vi "execute.vi"(8 "error in (no error)":errorcluster, 9 "ParameterString":string, 10 "ObjectCluster":T1, 11 "RoomLightCommand in":refnum<class "RoomLightCommand.lvclass">) -> (0 "error out":errorcluster, 2 "ObjectCluster Out":T1, 3 "RoomLightCommand out":refnum<class "RoomLightCommand.lvclass">)   [LabVIEW 2013, in "RoomLightCommand.lvclass"]
uses:
  RoomLightCommand.lvclass
  Command.lvclass/ObjectCluster.ctl
  AirCondition.lvclass/AirCondition.lvclass
  RoomLight.lvclass/RoomLight.lvclass
  OutDoorLight.lvclass/OutDoorLight.lvclass
  Television.lvclass/Television.lvclass
  Stereo.lvclass/Stereo.lvclass
  Command.lvclass/Command.lvclass
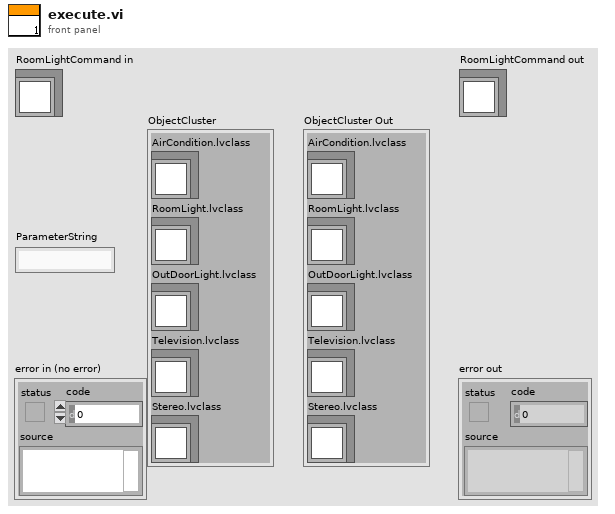
[diagram p1: front panel]
types:
  T1 = typedef "Command.lvclass/ObjectCluster.ctl" = cluster{"AirCondition.lvclass":refnum<class "AirCondition.lvclass">, "RoomLight.lvclass":refnum<class "RoomLight.lvclass">, "OutDoorLight.lvclass":refnum<class "OutDoorLight.lvclass">, "Television.lvclass":refnum<class "Television.lvclass">, "Stereo.lvclass":refnum<class "Stereo.lvclass">}
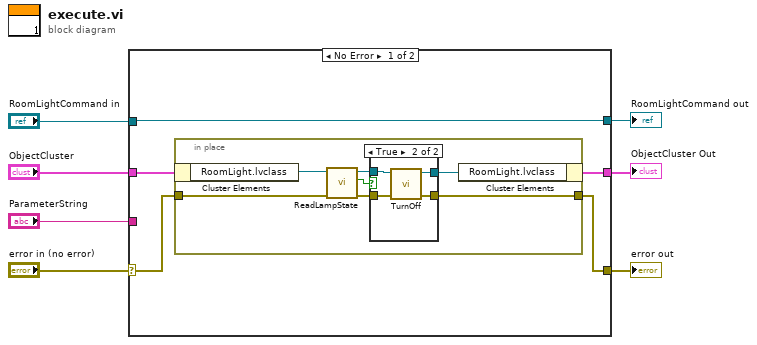
[diagram p0: block diagram]
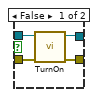
[diagram p2: hidden frame]
diagram:
  n1 = case shown="No Error" "error in (no error)" {
    selector: "error in (no error)" -> [w11 w28]
    tunnel: "ObjectCluster" -> [w12 w29]
    tunnel: "RoomLightCommand in" -> [w8 w30]
    tunnel: "ParameterString" -> [_ _]
    tunnel: [w10 w28] -> w3
    tunnel: [w9 w29] -> w2
    tunnel: [w8 w30] -> w1
    frame No Error {
      n2 = in-place {
        in-place-border: w11 -> [w14]
        in-place-border: [w13] -> w10
        n3 = in-place-cluster #1(w12) -> ("RoomLight.lvclass"=w16:refnum<class "RoomLight.lvclass">)
        n4 = call-dynamic "ReadLampState.vi"("error in (no error)"=w14, "RoomLight in"=w16) -> ("error out"=w17:errorcluster, "LampState"=w19:bool, "RoomLight out"=w18:refnum<class "RoomLight.lvclass">)  [unwired: 7 in]
        n5 = case shown="True" w19 {
          tunnel: w18 -> [w23 w27]
          tunnel: w17 -> [w21 w26]
          tunnel: [w22 w25] -> w15
          tunnel: [w20 w24] -> w13
          frame False {
            n6 = call-dynamic "TurnOn.vi"("error in (no error)"=w21, "RoomLight in"=w23) -> ("error out"=w20:errorcluster, "RoomLight out"=w22:refnum<class "RoomLight.lvclass">)  [unwired: 8 in]
          }
          frame True {
            n7 = call-dynamic "TurnOff.vi"("error in (no error)"=w26, "RoomLight in"=w27) -> ("error out"=w24:errorcluster, "RoomLight out"=w25:refnum<class "RoomLight.lvclass">)  [unwired: 8 in]
          }
        }
        n8 = in-place-cluster #1("RoomLight.lvclass"=w15) -> (w9:T1)
      }
    }
    frame Error {
    }
  }
  "error out" <- w3
  "RoomLightCommand out" <- w1
  "ObjectCluster Out" <- w2
